vi "indexToScriptIndex.vi"(8 "error in (no error)":errorcluster, 10 "sequencedIndex":i32, 11 "ScriptEventList in":refnum<class "ScriptEventList.lvclass">) -> (0 "error out":errorcluster, 2 "indexScriptEvent":i32, 3 "ScriptEventList out":refnum<class "ScriptEventList.lvclass">)   [LabVIEW 2009, in "Tools.lvlib" / "Scripting.lvlib" / "ScriptEventList.lvclass"]
uses:
  ScriptEventList.lvclass
  ScriptEventList.lvclass/ScriptEventList.ctl
  ScriptEvent.lvclass
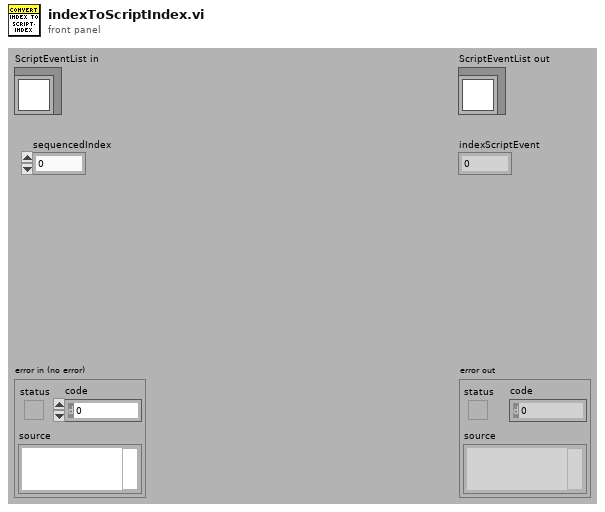
[diagram p1: front panel]
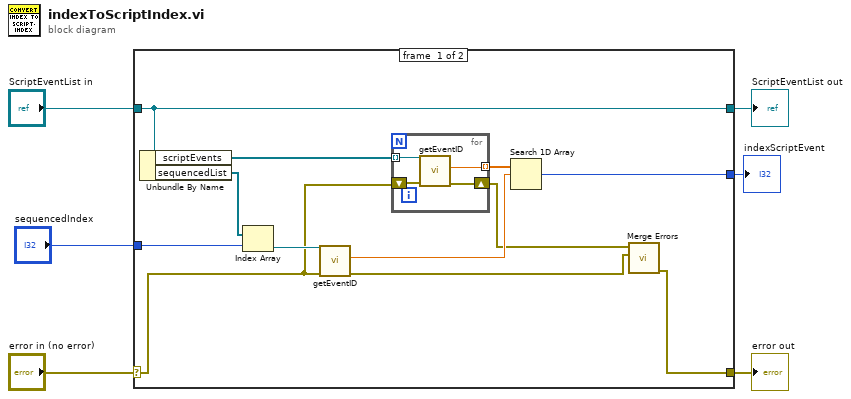
[diagram p0: block diagram]
diagram:
  n1 = case shown="No Error" "error in (no error)" {
    selector: "error in (no error)" -> [w14 w24]
    tunnel: [w7 w24] -> w5
    tunnel: [w18 w23] -> w3
    tunnel: "ScriptEventList in" -> [w18 w23]
    tunnel: "sequencedIndex" -> [w16 _]
    tunnel: [w10 _] -> w1
    frame #0 {
      n2 = Unbundle By Name(w18) -> ("scriptEvents"=w11:refnum<class "ScriptEvent.lvclass">[], "sequencedList"=w17:refnum<class "ScriptEvent.lvclass">[])
      n3 = Index Array(array=w17, index=w16) -> (element=w15:refnum<class "ScriptEvent.lvclass">)
      n4 = call "getEventID.vi"("error in (no error)"=w14, "ScriptEvent in"=w15) -> ("error out"=w8:errorcluster, "eventId"=w12:dbl)  [unwired: 7 in, 1 out]
      n5 = for {
        tunnel: w11 -> [w22] mode=indexing
        tunnel: [w20] -> w13 mode=indexing
        shift-right: [w19] -> w9
        shift-left: w14 -> [w21]
        n6 = call "getEventID.vi"("error in (no error)"=w21, "ScriptEvent in"=w22) -> ("error out"=w19:errorcluster, "eventId"=w20:dbl)  [unwired: 7 in, 1 out]
      }
      n7 = Search 1D Array(1D array=w13, element=w12) -> (index of element=w10:i32)  [unwired: 1 in]
      n8 = call <vilib>:"Merge Errors.vi"("error in 2 (no error)"=w8, "error in 1 (no error)"=w9) -> ("error out"=w7:errorcluster)  [unwired: 5 in]
    }
    frame #1 {
    }
  }
  "error out" <- w5
  "ScriptEventList out" <- w3
  "indexScriptEvent" <- w1
